vi "Setup for new units.vi"() -> (0 "Current Range":T1 {"Increment" format="%.2f"; "Maximum" format="%.2f"; "Minimum" format="%.2f"}, 1 "Current Slew Rate Caption":string, 2 "Current Setpoint Caption":string, 3 "Field Range":T1 {"Increment" format="%.2f"; "Maximum" format="%.2f"; "Minimum" format="%.2f"}, 4 "Field Slew Rate Caption":string, 5 "Field Setpoint Caption":string)   [LabVIEW 2020]
uses:
  PS Comm Globals.vi
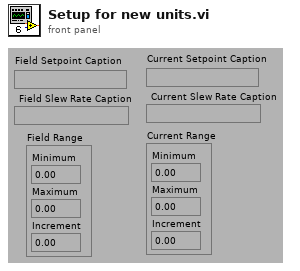
[diagram p1: front panel]
types:
  T1 = cluster{"Minimum":dbl, "Maximum":dbl, "Increment":dbl}
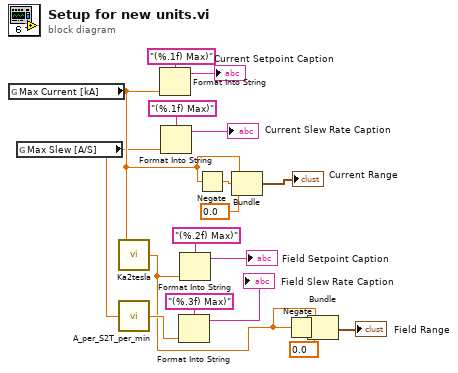
[diagram p0: block diagram]
diagram:
  n1 = global read "PS Comm Globals.vi" "Max Current [kA]"() -> (w17:dbl)
  n2 = global read "PS Comm Globals.vi" "Max Slew [A/S]"() -> (w3:dbl)
  n3 = call "Ka2tesla.vi"("Magnet Current [kA]"=w17) -> ("Field"=w5:dbl)  [unwired: 1 in]
  n4 = call "A_per_S2T_per_min.vi"("A/sec"=w3) -> ("T/min"=w9:dbl)
  n5 = Format Into String(format string="(%.1f) Max)", w17) -> (resulting string=→"Current Setpoint Caption":string)  [unwired: 2 in, 1 out]
  n6 = Format Into String(format string="(%.1f) Max)", w3) -> (resulting string=→"Current Slew Rate Caption":string)  [unwired: 2 in, 1 out]
  n7 = Format Into String(format string="(%.3f) Max)", w9) -> (resulting string=→"Field Slew Rate Caption":string)  [unwired: 2 in, 1 out]
  n8 = Format Into String(format string="(%.2f) Max)", w5) -> (resulting string=→"Field Setpoint Caption":string)  [unwired: 2 in, 1 out]
  n9 = Negate(x=w17) -> (-x=w18:dbl)
  n10 = Bundle("Max Current [kA]"=w17, w18, 0.0) -> (→"Current Range":cluster{"Max Current [kA]":dbl, dbl, dbl})  [unwired: 1 in]
  n11 = Negate(x=w5) -> (-x=w11:dbl)
  n12 = Bundle("Field"=w5, w11, 0.0) -> (→"Field Range":cluster{"Field":dbl, dbl, dbl})  [unwired: 1 in]
